vi "triquimejorado2.vi"() -> ()   [LabVIEW 2021]
panel:
  out "player X":dbl
  out "Player 0":dbl
  in  "Jump Button":bool
  out "appended array":u16[][](array[numeric])
  in  "OK Button":bool
  in  "x":bool
  in  "Ring 9":u16(ring)
  in  "Ring 8":u16(ring)
  in  "Ring 6":u16(ring)
  in  "Ring 5":u16(ring)
  in  "Ring 7":u16(ring)
  in  "Ring 4":u16(ring)
  in  "Ring 3":u16(ring)
  in  "Ring 2":u16(ring)
  in  "Ring":u16(ring)
  out "ocupado 9":bool
  out "ocupado 8":bool
  out "ocupado 7":bool
  out "ocupado 6":bool
  out "ocupado 5":bool
  out "ocupado 4":bool
  out "ocupado 3":bool
  out "ocupado 2":bool
  out "ocupado1":bool
  # "TRIQUI"
  # "TURNO"
  # "0"
  # "MARCADOR"
  # "OCUPACION"
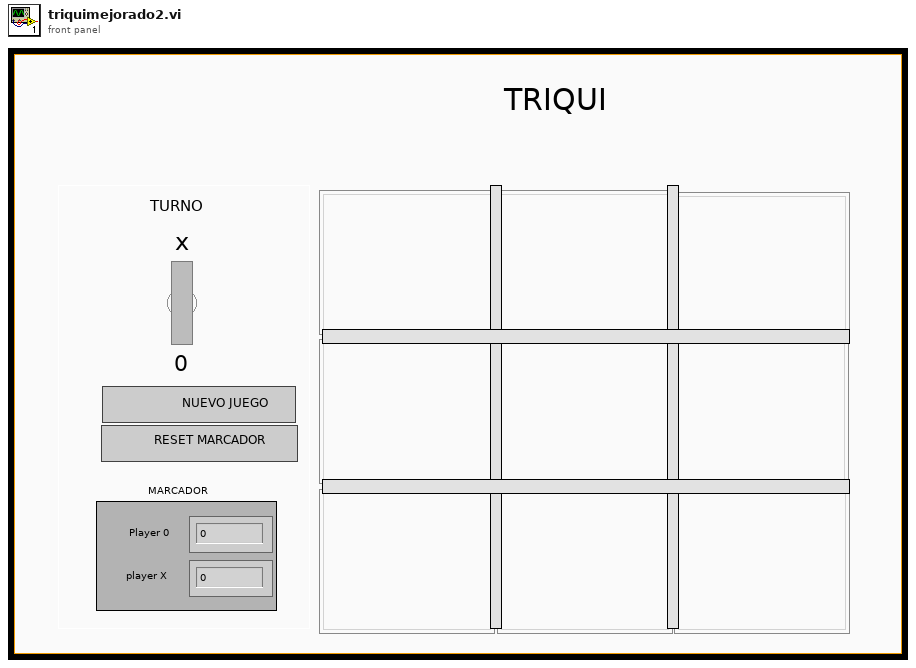
[diagram p1: front panel]
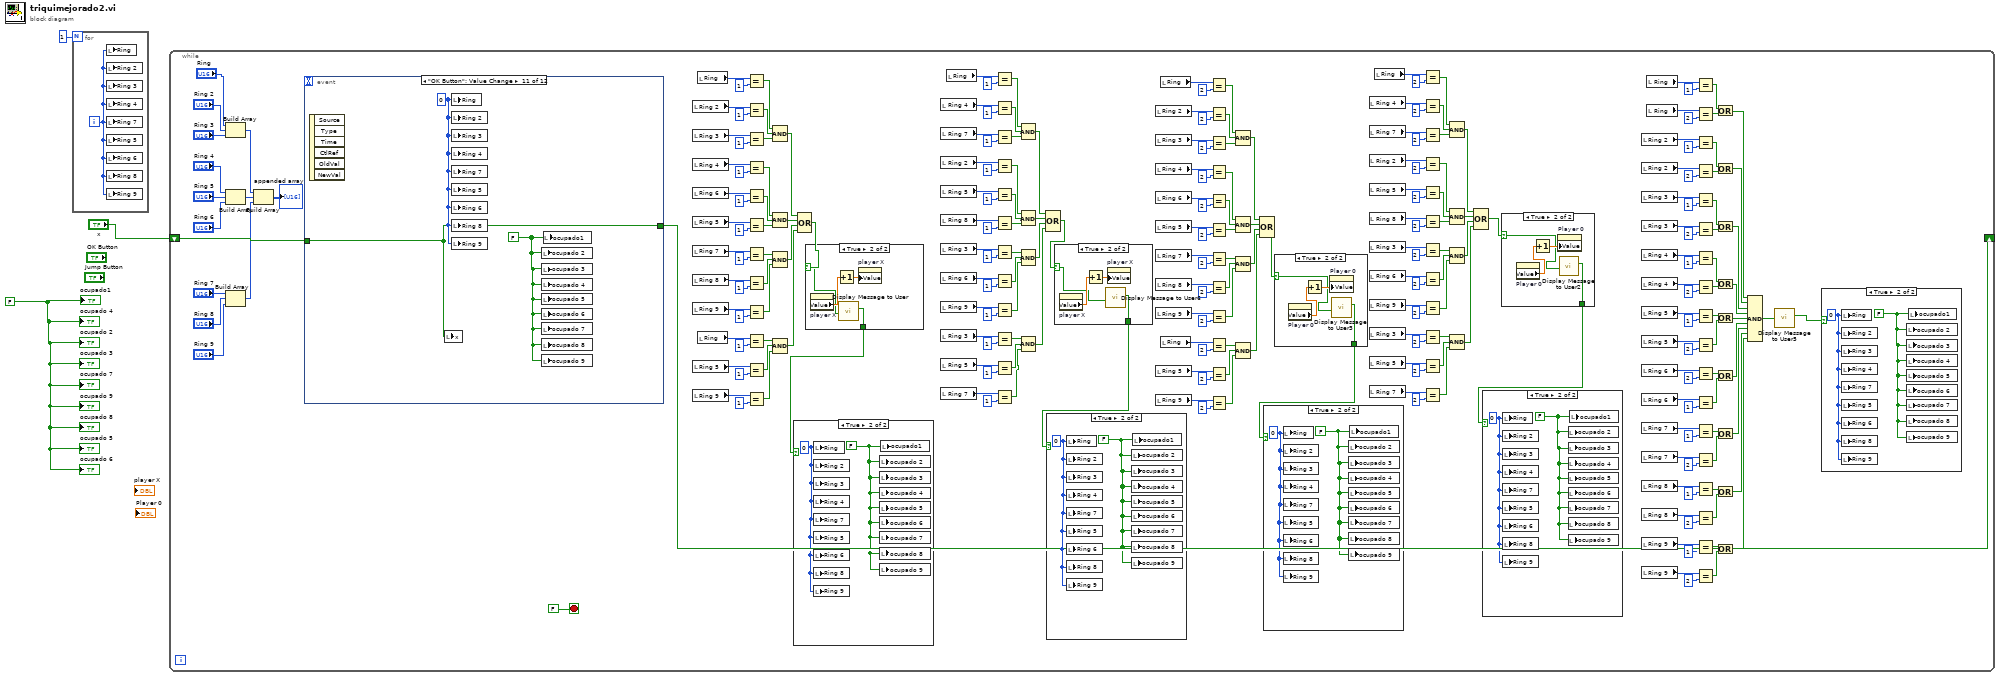
[diagram p0: block diagram]
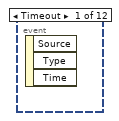
[diagram p11: hidden frame]
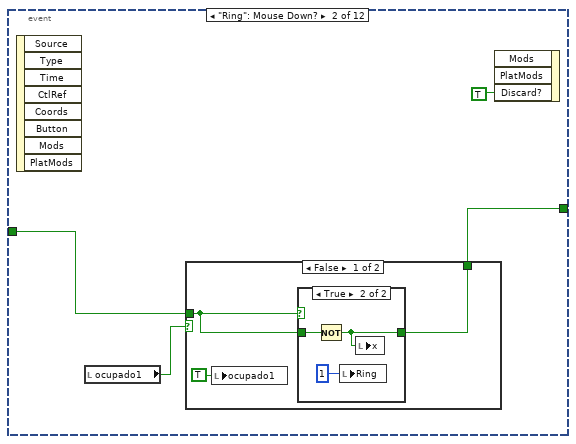
[diagram p12: hidden frame]
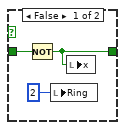
[diagram p13: hidden frame]
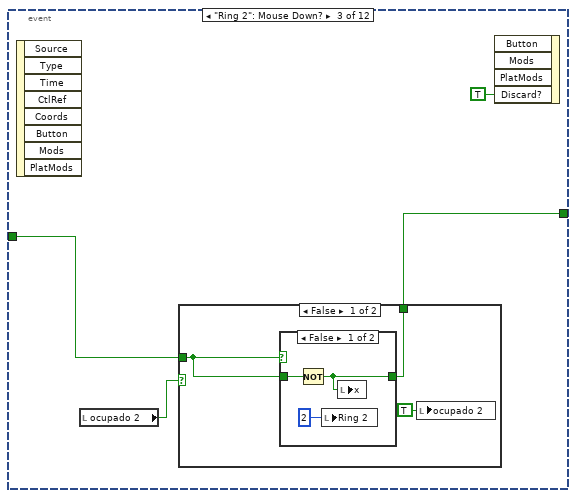
[diagram p15: hidden frame]
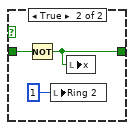
[diagram p16: hidden frame]
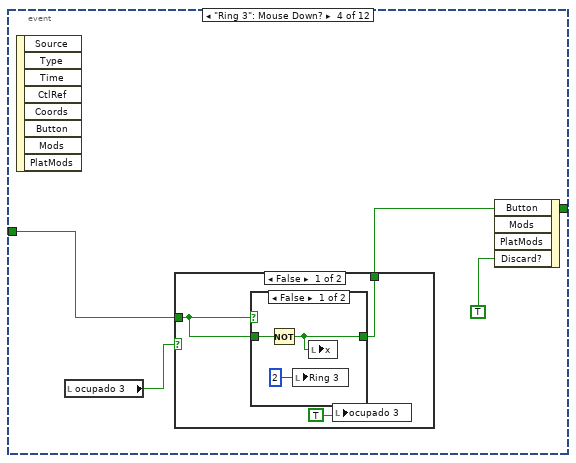
[diagram p18: hidden frame]
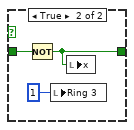
[diagram p19: hidden frame]
diagram:
  w1 = FALSE ("ocupado1")
  n1 = for {
    N: 1 -> [_]
    i -> [w4]
    n2 = local write "Ring"(w4) -> ()
    n3 = local write "Ring 2"(w4) -> ()
    n4 = local write "Ring 3"(w4) -> ()
    n5 = local write "Ring 4"(w4) -> ()
    n6 = local write "Ring 7"(w4) -> ()
    n7 = local write "Ring 5"(w4) -> ()
    n8 = local write "Ring 6"(w4) -> ()
    n9 = local write "Ring 8"(w4) -> ()
    n10 = local write "Ring 9"(w4) -> ()
  }
  n11 = while {
    shift-right: [w253] -> _
    shift-left: "x" -> [w252]
    stop <- FALSE stop-if-true
    n12 = Build Array("Ring", "Ring 2", "Ring 3") -> (w86:u16[])
    n13 = Build Array("Ring 4", "Ring 5", "Ring 6") -> (w85:u16[])
    n14 = Build Array("Ring 7", "Ring 8", "Ring 9") -> (w87:u16[])
    n15 = Build Array(w86, w85, w87) -> (→"appended array":u16[][])
    n16 = event shown="[10] \"OK Button\": Value Change" {
      selector: _ -> [_ _ _ _ _ _ _ _ _ _ _ _]
      dyn-events: _ -> [_ _ _ _ _ _ _ _ _ _ _ _]
      timeout: _ -> [_ _ _ _ _ _ _ _ _ _ _ _]
      tunnel: [_ w281 w295 w309 w323 w337 w351 w365 w379 w393 w407 _] -> w253
      tunnel: w252 -> [_ w282 w296 w310 w324 w338 w352 w366 w380 w394 w407 _]
      event Timeout {
        n17 = event-data() -> ()  [unwired: 1 in, 3 out]
      }
      event "Ring": Mouse Down? {
        n18 = event-data() -> ()  [unwired: 1 in, 8 out]
        n19 = local read "ocupado1"() -> (w280:bool)
        n20 = case shown="False" w280 {
          tunnel: w282 -> [w286 w293]
          tunnel: [w285 w293] -> w281
          frame False {
            n21 = local write "ocupado1"(TRUE ("ocupado1")) -> ()
            n22 = case shown="True" w286 {
              tunnel: [w288 w291] -> w285
              tunnel: w286 -> [w287 w290]
              frame False {
                n23 = Not(x=w287) -> (.not. x?=w288:bool)
                n24 = local write "Ring"(u16 2 ("Ring")) -> ()
                n25 = local write "x"(w288) -> ()
              }
              frame True {
                n26 = Not(x=w290) -> (.not. x?=w291:bool)
                n27 = local write "Ring"(u16 1 ("Ring")) -> ()
                n28 = local write "x"(w291) -> ()
              }
            }
          }
          frame True {
          }
        }
        n29 = event-data("Discard?"=TRUE) -> ()  [unwired: 3 in, 1 out]
      }
      event "Ring 2": Mouse Down? {
        n30 = event-data() -> ()  [unwired: 1 in, 8 out]
        n31 = local read "ocupado 2"() -> (w294:bool)
        n32 = case shown="False" w294 {
          tunnel: w296 -> [w300 w307]
          tunnel: [w299 w307] -> w295
          frame False {
            n33 = case shown="False" w300 {
              tunnel: w300 -> [w302 w305]
              tunnel: [w301 w304] -> w299
              frame False {
                n34 = Not(x=w302) -> (.not. x?=w301:bool)
                n35 = local write "Ring 2"(u16 2 ("Ring 2")) -> ()
                n36 = local write "x"(w301) -> ()
              }
              frame True {
                n37 = Not(x=w305) -> (.not. x?=w304:bool)
                n38 = local write "Ring 2"(u16 1 ("Ring 2")) -> ()
                n39 = local write "x"(w304) -> ()
              }
            }
            n40 = local write "ocupado 2"(TRUE ("ocupado 2")) -> ()
          }
          frame True {
          }
        }
        n41 = event-data("Discard?"=TRUE) -> ()  [unwired: 4 in, 1 out]
      }
      event "Ring 3": Mouse Down? {
        n42 = event-data() -> ()  [unwired: 1 in, 8 out]
        n43 = local read "ocupado 3"() -> (w308:bool)
        n44 = case shown="False" w308 {
          tunnel: w310 -> [w314 w321]
          tunnel: [w313 w321] -> w309
          frame False {
            n45 = case shown="False" w314 {
              tunnel: w314 -> [w316 w319]
              tunnel: [w315 w318] -> w313
              frame False {
                n46 = Not(x=w316) -> (.not. x?=w315:bool)
                n47 = local write "Ring 3"(u16 2 ("Ring 2")) -> ()
                n48 = local write "x"(w315) -> ()
              }
              frame True {
                n49 = Not(x=w319) -> (.not. x?=w318:bool)
                n50 = local write "Ring 3"(u16 1 ("Ring 2")) -> ()
                n51 = local write "x"(w318) -> ()
              }
            }
            n52 = local write "ocupado 3"(TRUE ("ocupado 3")) -> ()
          }
          frame True {
          }
        }
        n53 = event-data("Discard?"=TRUE) -> ()  [unwired: 4 in, 1 out]
      }
      event "Ring 4": Mouse Down? {
        n54 = event-data() -> ()  [unwired: 1 in, 8 out]
        n55 = local read "ocupado 4"() -> (w322:bool)
        n56 = case shown="False" w322 {
          tunnel: w324 -> [w328 w335]
          tunnel: [w327 w335] -> w323
          frame False {
            n57 = local write "ocupado 4"(TRUE ("ocupado 4")) -> ()
            n58 = case shown="False" w328 {
              tunnel: w328 -> [w330 w333]
              tunnel: [w329 w332] -> w327
              frame False {
                n59 = Not(x=w330) -> (.not. x?=w329:bool)
                n60 = local write "Ring 4"(u16 2 ("Ring 2")) -> ()
                n61 = local write "x"(w329) -> ()
              }
              frame True {
                n62 = Not(x=w333) -> (.not. x?=w332:bool)
                n63 = local write "Ring 4"(u16 1 ("Ring 2")) -> ()
                n64 = local write "x"(w332) -> ()
              }
            }
          }
          frame True {
          }
        }
        n65 = event-data("Discard?"=TRUE) -> ()  [unwired: 4 in, 1 out]
      }
      event "Ring 7": Mouse Down? {
        n66 = event-data() -> ()  [unwired: 1 in, 8 out]
        n67 = local read "ocupado 7"() -> (w336:bool)
        n68 = case shown="False" w336 {
          tunnel: w338 -> [w342 w349]
          tunnel: [w341 w349] -> w337
          frame False {
            n69 = local write "ocupado 7"(TRUE ("ocupado 7")) -> ()
            n70 = case shown="False" w342 {
              tunnel: w342 -> [w344 w347]
              tunnel: [w343 w346] -> w341
              frame False {
                n71 = Not(x=w344) -> (.not. x?=w343:bool)
                n72 = local write "Ring 7"(u16 2 ("Ring 2")) -> ()
                n73 = local write "x"(w343) -> ()
              }
              frame True {
                n74 = Not(x=w347) -> (.not. x?=w346:bool)
                n75 = local write "Ring 7"(u16 1 ("Ring 2")) -> ()
                n76 = local write "x"(w346) -> ()
              }
            }
          }
          frame True {
          }
        }
        n77 = event-data("Discard?"=TRUE) -> ()  [unwired: 4 in, 1 out]
      }
      event "Ring 5": Mouse Down? {
        n78 = event-data() -> ()  [unwired: 1 in, 8 out]
        n79 = local read "ocupado 5"() -> (w350:bool)
        n80 = case shown="False" w350 {
          tunnel: w352 -> [w356 w363]
          tunnel: [w355 w363] -> w351
          frame False {
            n81 = local write "ocupado 5"(TRUE ("ocupado 5")) -> ()
            n82 = case shown="True" w356 {
              tunnel: w356 -> [w358 w361]
              tunnel: [w357 w360] -> w355
              frame False {
                n83 = Not(x=w358) -> (.not. x?=w357:bool)
                n84 = local write "Ring 5"(u16 2 ("Ring 2")) -> ()
                n85 = local write "x"(w357) -> ()
              }
              frame True {
                n86 = Not(x=w361) -> (.not. x?=w360:bool)
                n87 = local write "Ring 5"(u16 1 ("Ring 2")) -> ()
                n88 = local write "x"(w360) -> ()
              }
            }
          }
          frame True {
          }
        }
        n89 = event-data("Discard?"=TRUE) -> ()  [unwired: 4 in, 1 out]
      }
      event "Ring 6": Mouse Down? {
        n90 = event-data() -> ()  [unwired: 1 in, 8 out]
        n91 = local read "ocupado 6"() -> (w364:bool)
        n92 = case shown="True" w364 {
          tunnel: w366 -> [w370 w377]
          tunnel: [w369 w377] -> w365
          frame False {
            n93 = local write "ocupado 6"(TRUE ("ocupado 6")) -> ()
            n94 = case shown="False" w370 {
              tunnel: w370 -> [w372 w375]
              tunnel: [w371 w374] -> w369
              frame False {
                n95 = Not(x=w372) -> (.not. x?=w371:bool)
                n96 = local write "Ring 6"(u16 2 ("Ring 2")) -> ()
                n97 = local write "x"(w371) -> ()
              }
              frame True {
                n98 = Not(x=w375) -> (.not. x?=w374:bool)
                n99 = local write "Ring 6"(u16 1 ("Ring 2")) -> ()
                n100 = local write "x"(w374) -> ()
              }
            }
          }
          frame True {
          }
        }
        n101 = event-data("Discard?"=TRUE) -> ()  [unwired: 4 in, 1 out]
      }
      event "Ring 8": Mouse Down? {
        n102 = event-data() -> ()  [unwired: 1 in, 8 out]
        n103 = local read "ocupado 8"() -> (w378:bool)
        n104 = case shown="False" w378 {
          tunnel: w380 -> [w384 w391]
          tunnel: [w383 w391] -> w379
          frame False {
            n105 = local write "ocupado 8"(TRUE ("ocupado 8")) -> ()
            n106 = case shown="False" w384 {
              tunnel: w384 -> [w386 w389]
              tunnel: [w385 w388] -> w383
              frame False {
                n107 = Not(x=w386) -> (.not. x?=w385:bool)
                n108 = local write "Ring 8"(u16 2 ("Ring 2")) -> ()
                n109 = local write "x"(w385) -> ()
              }
              frame True {
                n110 = Not(x=w389) -> (.not. x?=w388:bool)
                n111 = local write "Ring 8"(u16 1 ("Ring 2")) -> ()
                n112 = local write "x"(w388) -> ()
              }
            }
          }
          frame True {
          }
        }
        n113 = event-data("Discard?"=TRUE) -> ()  [unwired: 4 in, 1 out]
      }
      event "Ring 9": Mouse Down? {
        n114 = event-data() -> ()  [unwired: 1 in, 8 out]
        n115 = local read "ocupado 9"() -> (w392:bool)
        n116 = case shown="False" w392 {
          tunnel: w394 -> [w398 w405]
          tunnel: [w397 w405] -> w393
          frame False {
            n117 = local write "ocupado 9"(TRUE ("ocupado 9")) -> ()
            n118 = case shown="False" w398 {
              tunnel: w398 -> [w400 w403]
              tunnel: [w399 w402] -> w397
              frame False {
                n119 = Not(x=w400) -> (.not. x?=w399:bool)
                n120 = local write "Ring 9"(u16 2 ("Ring 2")) -> ()
                n121 = local write "x"(w399) -> ()
              }
              frame True {
                n122 = Not(x=w403) -> (.not. x?=w402:bool)
                n123 = local write "Ring 9"(u16 1 ("Ring 2")) -> ()
                n124 = local write "x"(w402) -> ()
              }
            }
          }
          frame True {
          }
        }
        n125 = event-data("Discard?"=TRUE) -> ()  [unwired: 4 in, 1 out]
      }
      event "OK Button": Value Change {
        w406 = FALSE ("ocupado1")
        w408 = u16 0 ("Ring")
        n126 = event-data() -> ()  [unwired: 1 in, 6 out]
        n127 = local write "x"(w407) -> ()
        n128 = local write "Ring"(w408) -> ()
        n129 = local write "Ring 2"(w408) -> ()
        n130 = local write "Ring 3"(w408) -> ()
        n131 = local write "Ring 4"(w408) -> ()
        n132 = local write "Ring 7"(w408) -> ()
        n133 = local write "Ring 5"(w408) -> ()
        n134 = local write "Ring 6"(w408) -> ()
        n135 = local write "Ring 8"(w408) -> ()
        n136 = local write "Ring 9"(w408) -> ()
        n137 = local write "ocupado 2"(w406) -> ()
        n138 = local write "ocupado 3"(w406) -> ()
        n139 = local write "ocupado 4"(w406) -> ()
        n140 = local write "ocupado 5"(w406) -> ()
        n141 = local write "ocupado 6"(w406) -> ()
        n142 = local write "ocupado 7"(w406) -> ()
        n143 = local write "ocupado 8"(w406) -> ()
        n144 = local write "ocupado 9"(w406) -> ()
        n145 = local write "ocupado1"(w406) -> ()
      }
      event "Jump Button": Value Change {
        n146 = event-data() -> ()  [unwired: 1 in, 6 out]
        n147 = property on="Player 0" class="DigNum (strict)"("Value"=0.0 ("Player 0")) -> ()  [unwired: 2 in, 2 out]
        n148 = property on="player X" class="DigNum (strict)"("Value"=0.0 ("player X")) -> ()  [unwired: 2 in, 2 out]
      }
    }
    n149 = local read "Ring 2"() -> (w249:u16)
    n150 = local read "Ring 3"() -> (w247:u16)
    n151 = local read "Ring 4"() -> (w236:u16)
    n152 = local read "Ring 6"() -> (w235:u16)
    n153 = local read "Ring 5"() -> (w234:u16)
    n154 = local read "Ring 7"() -> (w227:u16)
    n155 = local read "Ring 8"() -> (w226:u16)
    n156 = local read "Ring 9"() -> (w225:u16)
    n157 = local read "Ring 5"() -> (w220:u16)
    n158 = local read "Ring 9"() -> (w221:u16)
    n159 = local read "Ring"() -> (w251:u16)
    n160 = local read "Ring"() -> (w219:u16)
    n161 = Equal?(x=w251, y=u16 1) -> (x = y?=w245:bool)
    n162 = Equal?(x=w249, y=u16 1) -> (x = y?=w244:bool)
    n163 = Equal?(x=w247, y=u16 1) -> (x = y?=w243:bool)
    n164 = Equal?(x=w236, y=u16 1) -> (x = y?=w240:bool)
    n165 = Equal?(x=w235, y=u16 1) -> (x = y?=w241:bool)
    n166 = Equal?(x=w234, y=u16 1) -> (x = y?=w242:bool)
    n167 = Equal?(x=w227, y=u16 1) -> (x = y?=w230:bool)
    n168 = Equal?(x=w226, y=u16 1) -> (x = y?=w229:bool)
    n169 = Equal?(x=w225, y=u16 1) -> (x = y?=w228:bool)
    n170 = Equal?(x=w219, y=u16 1) -> (x = y?=w216:bool)
    n171 = Equal?(x=w220, y=u16 1) -> (x = y?=w217:bool)
    n172 = Equal?(x=w221, y=u16 1) -> (x = y?=w218:bool)
    n173 = Compound Arithmetic op=AND(w245, w244, w243) -> (w224:bool)
    n174 = Compound Arithmetic op=AND(w240, w241, w242) -> (w223:bool)
    n175 = Compound Arithmetic op=AND(w230, w229, w228) -> (w222:bool)
    n176 = Compound Arithmetic op=AND(w216, w217, w218) -> (w212:bool)
    n177 = Compound Arithmetic op=OR(w224, w223, w222, w212) -> (w14:bool)
    n178 = case shown="True" w14 {
      selector: w14 -> [_ w277]
      tunnel: [_ w276] -> w6
      frame False {
      }
      frame True {
        n179 = property on="player X" class="DigNum (strict)"() -> ("Value"=w278:dbl)  [unwired: 2 in, 2 out]
        n180 = Increment(x=w278) -> (x+1=w279:dbl)
        n181 = call "Display Message to User"("Enable"=w277) -> ("OK"=w276:bool)  [unwired: 9 in, 1 out]
        n182 = property on="player X" class="DigNum (strict)"("Value"=w279) -> ()  [unwired: 2 in, 2 out]
      }
    }
    n183 = case shown="True" w6 {
      frame False {
      }
      frame True {
        w262 = FALSE ("ocupado1")
        w263 = u16 0 ("Ring")
        n184 = local write "Ring"(w263) -> ()
        n185 = local write "Ring 2"(w263) -> ()
        n186 = local write "Ring 3"(w263) -> ()
        n187 = local write "Ring 4"(w263) -> ()
        n188 = local write "Ring 7"(w263) -> ()
        n189 = local write "Ring 5"(w263) -> ()
        n190 = local write "Ring 6"(w263) -> ()
        n191 = local write "Ring 8"(w263) -> ()
        n192 = local write "Ring 9"(w263) -> ()
        n193 = local write "ocupado 2"(w262) -> ()
        n194 = local write "ocupado 3"(w262) -> ()
        n195 = local write "ocupado 4"(w262) -> ()
        n196 = local write "ocupado 5"(w262) -> ()
        n197 = local write "ocupado 6"(w262) -> ()
        n198 = local write "ocupado 7"(w262) -> ()
        n199 = local write "ocupado 8"(w262) -> ()
        n200 = local write "ocupado 9"(w262) -> ()
        n201 = local write "ocupado1"(w262) -> ()
      }
    }
    n202 = local read "Ring 4"() -> (w175:u16)
    n203 = local read "Ring 7"() -> (w177:u16)
    n204 = local read "Ring 2"() -> (w188:u16)
    n205 = local read "Ring 5"() -> (w189:u16)
    n206 = local read "Ring 8"() -> (w190:u16)
    n207 = local read "Ring 3"() -> (w197:u16)
    n208 = local read "Ring 6"() -> (w198:u16)
    n209 = local read "Ring 9"() -> (w199:u16)
    n210 = local read "Ring 3"() -> (w205:u16)
    n211 = local read "Ring 5"() -> (w204:u16)
    n212 = local read "Ring 7"() -> (w203:u16)
    n213 = local read "Ring"() -> (w173:u16)
    n214 = Equal?(x=w173, y=u16 1) -> (x = y?=w179:bool)
    n215 = Equal?(x=w175, y=u16 1) -> (x = y?=w180:bool)
    n216 = Equal?(x=w177, y=u16 1) -> (x = y?=w181:bool)
    n217 = Equal?(x=w188, y=u16 1) -> (x = y?=w184:bool)
    n218 = Equal?(x=w189, y=u16 1) -> (x = y?=w183:bool)
    n219 = Equal?(x=w190, y=u16 1) -> (x = y?=w182:bool)
    n220 = Equal?(x=w197, y=u16 1) -> (x = y?=w194:bool)
    n221 = Equal?(x=w198, y=u16 1) -> (x = y?=w195:bool)
    n222 = Equal?(x=w199, y=u16 1) -> (x = y?=w196:bool)
    n223 = Equal?(x=w205, y=u16 1) -> (x = y?=w207:bool)
    n224 = Equal?(x=w204, y=u16 1) -> (x = y?=w206:bool)
    n225 = Equal?(x=w203, y=u16 1) -> (x = y?=w10:bool)
    n226 = Compound Arithmetic op=AND(w179, w180, w181) -> (w200:bool)
    n227 = Compound Arithmetic op=AND(w184, w183, w182) -> (w201:bool)
    n228 = Compound Arithmetic op=AND(w194, w195, w196) -> (w202:bool)
    n229 = Compound Arithmetic op=AND(w207, w206, w10) -> (w211:bool)
    n230 = Compound Arithmetic op=OR(w200, w201, w202, w211) -> (w13:bool)
    n231 = case shown="True" w13 {
      selector: w13 -> [_ w273]
      tunnel: [_ w272] -> w9
      frame False {
      }
      frame True {
        n232 = property on="player X" class="DigNum (strict)"() -> ("Value"=w274:dbl)  [unwired: 2 in, 2 out]
        n233 = Increment(x=w274) -> (x+1=w275:dbl)
        n234 = call "Display Message to User6"("Enable"=w273) -> ("OK"=w272:bool)  [unwired: 9 in, 1 out]
        n235 = property on="player X" class="DigNum (strict)"("Value"=w275) -> ()  [unwired: 2 in, 2 out]
      }
    }
    n236 = case shown="True" w9 {
      frame False {
      }
      frame True {
        w260 = FALSE ("ocupado1")
        w261 = u16 0 ("Ring")
        n237 = local write "Ring"(w261) -> ()
        n238 = local write "Ring 2"(w261) -> ()
        n239 = local write "Ring 3"(w261) -> ()
        n240 = local write "Ring 4"(w261) -> ()
        n241 = local write "Ring 7"(w261) -> ()
        n242 = local write "Ring 5"(w261) -> ()
        n243 = local write "Ring 6"(w261) -> ()
        n244 = local write "Ring 8"(w261) -> ()
        n245 = local write "Ring 9"(w261) -> ()
        n246 = local write "ocupado 2"(w260) -> ()
        n247 = local write "ocupado 3"(w260) -> ()
        n248 = local write "ocupado 4"(w260) -> ()
        n249 = local write "ocupado 5"(w260) -> ()
        n250 = local write "ocupado 6"(w260) -> ()
        n251 = local write "ocupado 7"(w260) -> ()
        n252 = local write "ocupado 8"(w260) -> ()
        n253 = local write "ocupado 9"(w260) -> ()
        n254 = local write "ocupado1"(w260) -> ()
      }
    }
    n255 = local read "Ring 2"() -> (w95:u16)
    n256 = local read "Ring 3"() -> (w97:u16)
    n257 = local read "Ring 4"() -> (w108:u16)
    n258 = local read "Ring 6"() -> (w109:u16)
    n259 = local read "Ring 5"() -> (w110:u16)
    n260 = local read "Ring 7"() -> (w117:u16)
    n261 = local read "Ring 8"() -> (w118:u16)
    n262 = local read "Ring 9"() -> (w119:u16)
    n263 = local read "Ring 5"() -> (w124:u16)
    n264 = local read "Ring 9"() -> (w123:u16)
    n265 = local read "Ring"() -> (w93:u16)
    n266 = local read "Ring"() -> (w125:u16)
    n267 = Equal?(x=w93, y=u16 2) -> (x = y?=w99:bool)
    n268 = Equal?(x=w95, y=u16 2) -> (x = y?=w100:bool)
    n269 = Equal?(x=w97, y=u16 2) -> (x = y?=w101:bool)
    n270 = Equal?(x=w108, y=u16 2) -> (x = y?=w104:bool)
    n271 = Equal?(x=w109, y=u16 2) -> (x = y?=w103:bool)
    n272 = Equal?(x=w110, y=u16 2) -> (x = y?=w102:bool)
    n273 = Equal?(x=w117, y=u16 2) -> (x = y?=w114:bool)
    n274 = Equal?(x=w118, y=u16 2) -> (x = y?=w115:bool)
    n275 = Equal?(x=w119, y=u16 2) -> (x = y?=w116:bool)
    n276 = Equal?(x=w125, y=u16 2) -> (x = y?=w128:bool)
    n277 = Equal?(x=w124, y=u16 2) -> (x = y?=w127:bool)
    n278 = Equal?(x=w123, y=u16 2) -> (x = y?=w126:bool)
    n279 = Compound Arithmetic op=AND(w99, w100, w101) -> (w120:bool)
    n280 = Compound Arithmetic op=AND(w104, w103, w102) -> (w121:bool)
    n281 = Compound Arithmetic op=AND(w114, w115, w116) -> (w122:bool)
    n282 = Compound Arithmetic op=AND(w128, w127, w126) -> (w132:bool)
    n283 = Compound Arithmetic op=OR(w120, w121, w122, w132) -> (w12:bool)
    n284 = case shown="True" w12 {
      selector: w12 -> [_ w269]
      tunnel: [_ w268] -> w8
      frame False {
      }
      frame True {
        n285 = property on="Player 0" class="DigNum (strict)"() -> ("Value"=w270:dbl)  [unwired: 2 in, 2 out]
        n286 = Increment(x=w270) -> (x+1=w271:dbl)
        n287 = property on="Player 0" class="DigNum (strict)"("Value"=w271) -> ()  [unwired: 2 in, 2 out]
        n288 = call "Display Message to User3"("Enable"=w269) -> ("OK"=w268:bool)  [unwired: 9 in, 1 out]
      }
    }
    n289 = case shown="True" w8 {
      frame False {
      }
      frame True {
        w258 = FALSE ("ocupado1")
        w259 = u16 0 ("Ring")
        n290 = local write "Ring"(w259) -> ()
        n291 = local write "Ring 2"(w259) -> ()
        n292 = local write "Ring 3"(w259) -> ()
        n293 = local write "Ring 4"(w259) -> ()
        n294 = local write "Ring 7"(w259) -> ()
        n295 = local write "Ring 5"(w259) -> ()
        n296 = local write "Ring 6"(w259) -> ()
        n297 = local write "Ring 8"(w259) -> ()
        n298 = local write "Ring 9"(w259) -> ()
        n299 = local write "ocupado 2"(w258) -> ()
        n300 = local write "ocupado 3"(w258) -> ()
        n301 = local write "ocupado 4"(w258) -> ()
        n302 = local write "ocupado 5"(w258) -> ()
        n303 = local write "ocupado 6"(w258) -> ()
        n304 = local write "ocupado 7"(w258) -> ()
        n305 = local write "ocupado 8"(w258) -> ()
        n306 = local write "ocupado 9"(w258) -> ()
        n307 = local write "ocupado1"(w258) -> ()
      }
    }
    n308 = local read "Ring 4"() -> (w170:u16)
    n309 = local read "Ring 7"() -> (w168:u16)
    n310 = local read "Ring 2"() -> (w157:u16)
    n311 = local read "Ring 5"() -> (w156:u16)
    n312 = local read "Ring 8"() -> (w155:u16)
    n313 = local read "Ring 3"() -> (w148:u16)
    n314 = local read "Ring 6"() -> (w147:u16)
    n315 = local read "Ring 9"() -> (w146:u16)
    n316 = local read "Ring 3"() -> (w140:u16)
    n317 = local read "Ring 5"() -> (w141:u16)
    n318 = local read "Ring 7"() -> (w142:u16)
    n319 = local read "Ring"() -> (w172:u16)
    n320 = Equal?(x=w172, y=u16 2) -> (x = y?=w166:bool)
    n321 = Equal?(x=w170, y=u16 2) -> (x = y?=w165:bool)
    n322 = Equal?(x=w168, y=u16 2) -> (x = y?=w164:bool)
    n323 = Equal?(x=w157, y=u16 2) -> (x = y?=w161:bool)
    n324 = Equal?(x=w156, y=u16 2) -> (x = y?=w162:bool)
    n325 = Equal?(x=w155, y=u16 2) -> (x = y?=w163:bool)
    n326 = Equal?(x=w148, y=u16 2) -> (x = y?=w151:bool)
    n327 = Equal?(x=w147, y=u16 2) -> (x = y?=w150:bool)
    n328 = Equal?(x=w146, y=u16 2) -> (x = y?=w149:bool)
    n329 = Equal?(x=w140, y=u16 2) -> (x = y?=w137:bool)
    n330 = Equal?(x=w141, y=u16 2) -> (x = y?=w138:bool)
    n331 = Equal?(x=w142, y=u16 2) -> (x = y?=w139:bool)
    n332 = Compound Arithmetic op=AND(w166, w165, w164) -> (w145:bool)
    n333 = Compound Arithmetic op=AND(w161, w162, w163) -> (w144:bool)
    n334 = Compound Arithmetic op=AND(w151, w150, w149) -> (w143:bool)
    n335 = Compound Arithmetic op=AND(w137, w138, w139) -> (w133:bool)
    n336 = Compound Arithmetic op=OR(w145, w144, w143, w133) -> (w11:bool)
    n337 = case shown="True" w11 {
      selector: w11 -> [_ w265]
      tunnel: [_ w264] -> w7
      frame False {
      }
      frame True {
        n338 = property on="Player 0" class="DigNum (strict)"() -> ("Value"=w266:dbl)  [unwired: 2 in, 2 out]
        n339 = Increment(x=w266) -> (x+1=w267:dbl)
        n340 = property on="Player 0" class="DigNum (strict)"("Value"=w267) -> ()  [unwired: 2 in, 2 out]
        n341 = call "Display Message to User2"("Enable"=w265) -> ("OK"=w264:bool)  [unwired: 9 in, 1 out]
      }
    }
    n342 = case shown="True" w7 {
      frame False {
      }
      frame True {
        w256 = FALSE ("ocupado1")
        w257 = u16 0 ("Ring")
        n343 = local write "Ring"(w257) -> ()
        n344 = local write "Ring 2"(w257) -> ()
        n345 = local write "Ring 3"(w257) -> ()
        n346 = local write "Ring 4"(w257) -> ()
        n347 = local write "Ring 7"(w257) -> ()
        n348 = local write "Ring 5"(w257) -> ()
        n349 = local write "Ring 6"(w257) -> ()
        n350 = local write "Ring 8"(w257) -> ()
        n351 = local write "Ring 9"(w257) -> ()
        n352 = local write "ocupado 2"(w256) -> ()
        n353 = local write "ocupado 3"(w256) -> ()
        n354 = local write "ocupado 4"(w256) -> ()
        n355 = local write "ocupado 5"(w256) -> ()
        n356 = local write "ocupado 6"(w256) -> ()
        n357 = local write "ocupado 7"(w256) -> ()
        n358 = local write "ocupado 8"(w256) -> ()
        n359 = local write "ocupado 9"(w256) -> ()
        n360 = local write "ocupado1"(w256) -> ()
      }
    }
    n361 = local read "Ring 2"() -> (w71:u16)
    n362 = local read "Ring 2"() -> (w74:u16)
    n363 = local read "Ring 3"() -> (w70:u16)
    n364 = local read "Ring 3"() -> (w67:u16)
    n365 = local read "Ring 4"() -> (w63:u16)
    n366 = local read "Ring 4"() -> (w66:u16)
    n367 = local read "Ring 5"() -> (w62:u16)
    n368 = local read "Ring 5"() -> (w59:u16)
    n369 = local read "Ring 6"() -> (w58:u16)
    n370 = local read "Ring 6"() -> (w55:u16)
    n371 = local read "Ring 7"() -> (w54:u16)
    n372 = local read "Ring 7"() -> (w51:u16)
    n373 = local read "Ring 8"() -> (w47:u16)
    n374 = local read "Ring 8"() -> (w50:u16)
    n375 = local read "Ring 9"() -> (w46:u16)
    n376 = local read "Ring 9"() -> (w43:u16)
    n377 = local read "Ring"() -> (w78:u16)
    n378 = local read "Ring"() -> (w75:u16)
    n379 = Equal?(x=w78, y=u16 1) -> (x = y?=w42:bool)
    n380 = Equal?(x=w75, y=u16 2) -> (x = y?=w41:bool)
    n381 = Equal?(x=w71, y=u16 1) -> (x = y?=w40:bool)
    n382 = Equal?(x=w74, y=u16 2) -> (x = y?=w39:bool)
    n383 = Equal?(x=w70, y=u16 1) -> (x = y?=w36:bool)
    n384 = Equal?(x=w67, y=u16 2) -> (x = y?=w35:bool)
    n385 = Equal?(x=w63, y=u16 1) -> (x = y?=w34:bool)
    n386 = Equal?(x=w66, y=u16 2) -> (x = y?=w33:bool)
    n387 = Equal?(x=w62, y=u16 1) -> (x = y?=w32:bool)
    n388 = Equal?(x=w59, y=u16 2) -> (x = y?=w31:bool)
    n389 = Equal?(x=w58, y=u16 2) -> (x = y?=w30:bool)
    n390 = Equal?(x=w55, y=u16 1) -> (x = y?=w38:bool)
    n391 = Equal?(x=w54, y=u16 1) -> (x = y?=w29:bool)
    n392 = Equal?(x=w51, y=u16 2) -> (x = y?=w37:bool)
    n393 = Equal?(x=w47, y=u16 1) -> (x = y?=w28:bool)
    n394 = Equal?(x=w50, y=u16 2) -> (x = y?=w27:bool)
    n395 = Equal?(x=w46, y=u16 1) -> (x = y?=w26:bool)
    n396 = Equal?(x=w43, y=u16 2) -> (x = y?=w25:bool)
    n397 = Or(x=w42, y=w41) -> (x .or. y?=w24:bool)
    n398 = Or(x=w40, y=w39) -> (x .or. y?=w23:bool)
    n399 = Or(x=w36, y=w35) -> (x .or. y?=w22:bool)
    n400 = Or(x=w34, y=w33) -> (x .or. y?=w21:bool)
    n401 = Or(x=w32, y=w31) -> (x .or. y?=w20:bool)
    n402 = Or(x=w30, y=w38) -> (x .or. y?=w19:bool)
    n403 = Or(x=w29, y=w37) -> (x .or. y?=w18:bool)
    n404 = Or(x=w28, y=w27) -> (x .or. y?=w17:bool)
    n405 = Or(x=w26, y=w25) -> (x .or. y?=w16:bool)
    n406 = Compound Arithmetic op=AND(w24, w23, w22, w21, w20, w19, w18, w17, w16) -> (w15:bool)
    n407 = call "Display Message to User5"("Enable"=w15) -> ("OK"=w5:bool)  [unwired: 9 in, 1 out]
    n408 = case shown="True" w5 {
      frame False {
      }
      frame True {
        w254 = FALSE ("ocupado1")
        w255 = u16 0 ("Ring")
        n409 = local write "Ring"(w255) -> ()
        n410 = local write "Ring 2"(w255) -> ()
        n411 = local write "Ring 3"(w255) -> ()
        n412 = local write "Ring 4"(w255) -> ()
        n413 = local write "Ring 7"(w255) -> ()
        n414 = local write "Ring 5"(w255) -> ()
        n415 = local write "Ring 6"(w255) -> ()
        n416 = local write "Ring 8"(w255) -> ()
        n417 = local write "Ring 9"(w255) -> ()
        n418 = local write "ocupado 2"(w254) -> ()
        n419 = local write "ocupado 3"(w254) -> ()
        n420 = local write "ocupado 4"(w254) -> ()
        n421 = local write "ocupado 5"(w254) -> ()
        n422 = local write "ocupado 6"(w254) -> ()
        n423 = local write "ocupado 7"(w254) -> ()
        n424 = local write "ocupado 8"(w254) -> ()
        n425 = local write "ocupado 9"(w254) -> ()
        n426 = local write "ocupado1"(w254) -> ()
      }
    }
  }
  "ocupado1" <- w1
  "ocupado 2" <- w1
  "ocupado 3" <- w1
  "ocupado 4" <- w1
  "ocupado 5" <- w1
  "ocupado 6" <- w1
  "ocupado 7" <- w1
  "ocupado 8" <- w1
  "ocupado 9" <- w1
